vi "CRM-Config (PXI).vi"(7 "Path":path, 8 "error in (no error)":errorcluster, 9 "AI Channels":i32[](array[numeric]), 10 "Num AI pts":i32, 11 "Sampling Rate (Hz)":dbl=20000.0) -> (0 "error out":errorcluster, 1 "Magnitude array":dbl[](array[numeric]), 3 "Freq resol (Hz)":dbl)   [LabVIEW 2020]
uses:
  epl-vi-lib/PXI DAQ VIs/DAQ Engine VIs/PXI Globals.vi
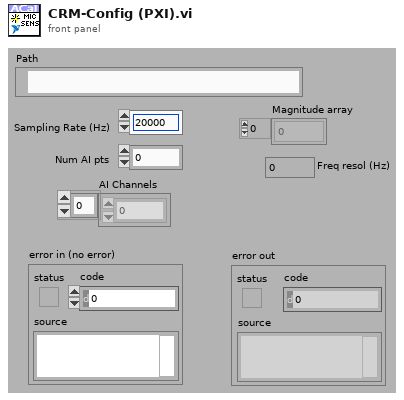
[diagram p1: front panel]
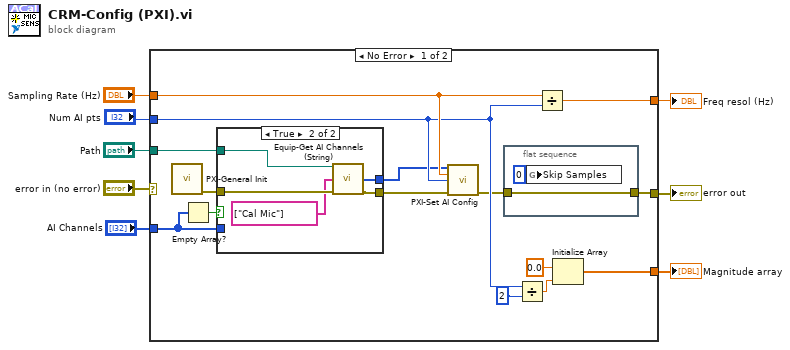
[diagram p0: block diagram]
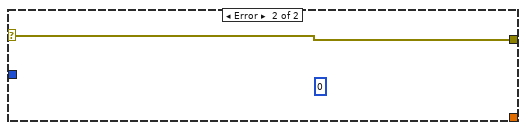
[diagram p3: hidden frame]
diagram:
  n1 = case shown="No Error" "error in (no error)" {
    selector: "error in (no error)" -> [_ w33]
    tunnel: [w15 w33] -> w7
    tunnel: "Num AI pts" -> [w17 _]
    tunnel: "Sampling Rate (Hz)" -> [w18 _]
    tunnel: [w23 _] -> w4
    tunnel: [w19 _] -> w3
    tunnel: "AI Channels" -> [w12 _]
    tunnel: "Path" -> [w10 _]
    frame No Error {
      n2 = call "PXI-General Init.vi"() -> ("error out"=w14:errorcluster)  [unwired: 11 in]
      n3 = Empty Array?(array=w12) -> (empty?=w11:bool)
      n4 = case shown="True" w11 {
        tunnel: w14 -> [w24 w30]
        tunnel: [w24 w29] -> w13
        tunnel: [w25 w28] -> w9
        tunnel: w12 -> [w25 _]
        tunnel: w10 -> [_ w26]
        frame False {
        }
        frame True {
          n5 = call "Equip-Get AI Channels (String).vi"("Path"=w26, "Inputs"=string[] ["Cal Mic"], "error in (no error)"=w30) -> ("AI Channels"=w28:i32[], "error out"=w29:errorcluster)  [unwired: 11 in]
        }
      }
      n6 = call "PXI-Set AI Config.vi"("AI Channels"=w9, "Sampling Rate (Hz)"=w18, "Buffer Size"=w17, "error in (no error)"=w13) -> ("error out"=w16:errorcluster)  [unwired: 11 in]
      n7 = flat-sequence {
        tunnel: w16 -> [w32]
        tunnel: [w32] -> w15
        frame #0 {
          n8 = global write "PXI Globals.vi" "Skip Samples"(0 ("Skip Samples")) -> ()
        }
      }
      n9 = Divide(x=w17, y=2) -> (x/y=w21:dbl)
      n10 = Divide(x=w18, y=w17) -> (x/y=w23:dbl)
      n11 = Initialize Array(0.0 ("element"), w21) -> (w19:dbl[])
    }
    frame Error {
      (unwired) 0
    }
  }
  "error out" <- w7
  "Freq resol (Hz)" <- w4
  "Magnitude array" <- w3
